vi "gRPC Stream Performance Test.vi"() -> ()   [LabVIEW 2021]
uses:
  streamtest_server/RPC Messages/streamtest_StreamData.ctl
  streamtest_client/RPC Messages/streamtest_StreamData.ctl
  <vilib>/gRPC/LabVIEW gRPC Servicer/Servicer/Servicer.lvclass/Servicer.ctl
  streamtest_server/RPC Service/stream/stream.lvclass
  <vilib>/Platform/TimedLoop/XDataNode/timing_clust.ctl
  <vilib>/Platform/TimedLoop/XDataNode/nitl_modes.ctl
  <vilib>/Platform/TimedLoop/XDataNode/wakeup.ctl
  streamtest_server/RPC Service/stream/stream.lvclass/stream.ctl
  6ba0af29-652a-47d8-b42d-4f43e62654bc.vi
  4033fe76-a443-4ae7-8d99-8cf937cf737c.vi
  <vilib>/gRPC/LabVIEW gRPC Library/Shared/TranslateGrpcError.vi
  grpc perf attempts/_Client obtain occurance.vi
  <vilib>/gRPC/LabVIEW gRPC Library/Server API/Server/Get Server DLL Path.vi
  <vilib>/Utility/error.llb/Error Cluster From Error Code.vi
  <vilib>/Platform/TimedLoop/XDataNode/XDataNode.xnode
  <vilib>/Platform/TimedLoop/XDataNode/XDNodeRunTimeDep.lvlib
  <vilib>/gRPC/LabVIEW gRPC Servicer/Servicer/Servicer.lvclass
  streamtest_server/streamtest_server.lvlib
  streamtest_client/streamtest_client.lvlib
  <vilib>/gRPC/LabVIEW gRPC Library/grpc-lvsupport-release.lvlib
panel:
  out "error out 4":errorcluster
  out "pass 2":bool
  out "avg stream":dbl
  out "Response Data 2":T1
  out "error out 3":errorcluster
  out "Response Data":T1
  out "error out 2":errorcluster
  out "output cluster":T2
  in  "stop":bool
  out "Listening Port":i32
  in  "Server Address":string="localhost:50051"
  in  "Server Certificate File (.crt)":path
  in  "Server Key File (.key)":path
  out "max stream":dbl
  out "pass":bool
  out "error out":errorcluster
  # "This test should be run on RT.  It stresses the communications by constantly creating resource contraints with the low priority sender and the high priority loop. On Windows the priority of the loops cannot be set."
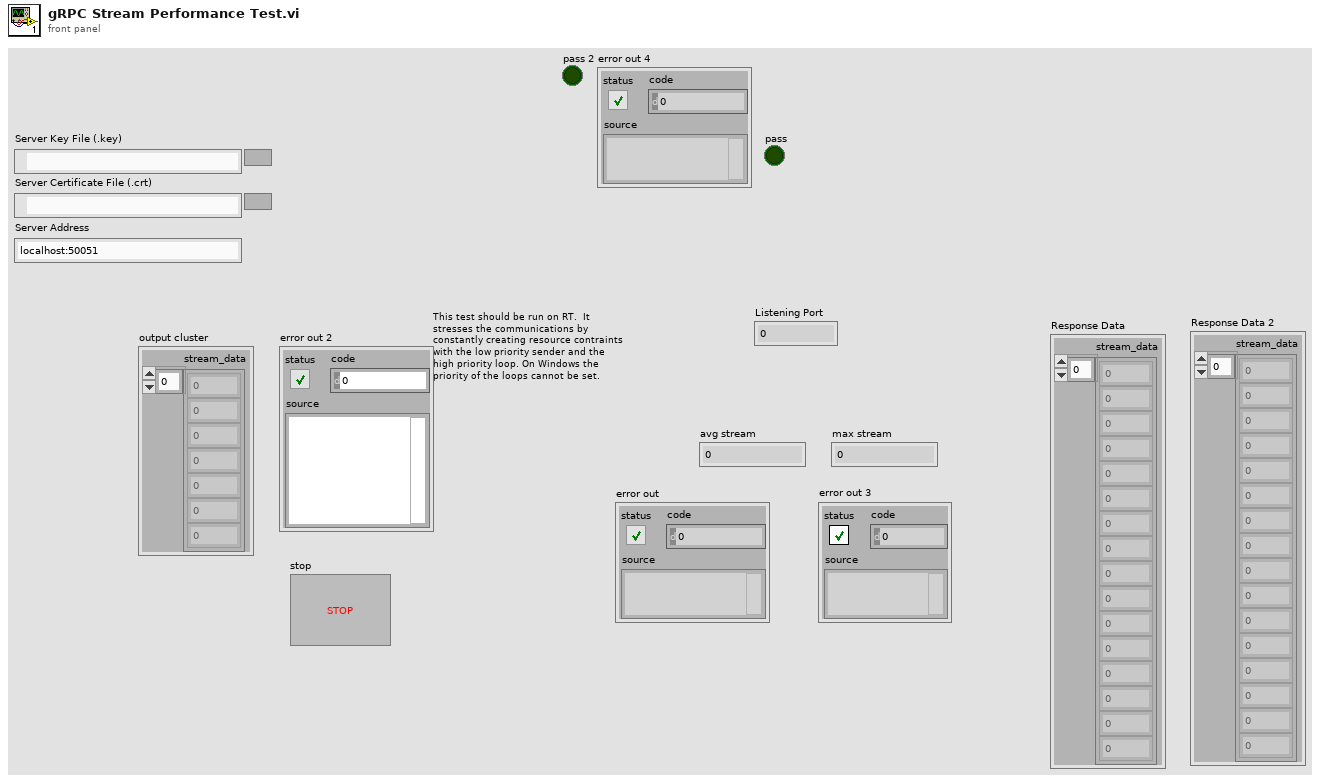
[diagram p1: front panel]
types:
  T1 = typedef "streamtest_client.lvlib/streamtest_StreamData.ctl" = cluster{"stream_data":u8[]}
  T2 = typedef "streamtest_server.lvlib/streamtest_StreamData.ctl" = cluster{"stream_data":u8[]}
  T3 = typedef "grpc-lvsupport-release.lvlib/grpcId.ctl" = u64
  T4 = typedef "Call ID.ctl" = cluster{"Call Id":T3, "occurrence":refnum<k4>}
  T5 = typedef "XDNodeRunTimeDep.lvlib/timing_clust.ctl" = cluster{"Expected End [f-1]":u64, "Actual End [f-1]":u64, "Finished Late? [f-1]":bool, "Expected End [i-1]":u64, "Actual End [i-1]":u64, "Finished Late? [i-1]":bool, "Expected Start [i]":u64, "Actual Start [i]":u64, "Expected Start [f]":u64, "Actual Start [f]":u64, "Source Name":string, "Structure Name":string, "Period":i64, "Deadline":i64, "Offset":i64, "Start":i64, "Priority":i32, "Timeout":i32, "Mode":T6, "Wakeup Reason":T7, "Error":errorcluster, "Source Type":string, "Secondary Source Type":string, "Global End Time":u64, "Global Start Time":u64, "Frame Duration":u64, "Iteration Duration":u64, "Assigned CPU":i32, "I/O Scan Engine Mode":u32}
  T6 = typedef "XDNodeRunTimeDep.lvlib/nitl_modes.ctl" = enum32{"No Change", "Process missed periods, maintain original phase", "Discard missed periods, maintain original phase", "Process missed periods, ignore original phase", "Discard missed periods, ignore original phase"}
  T7 = typedef "XDNodeRunTimeDep.lvlib/wakeup.ctl" = enum32{"Normal", "Aborted", "Asynchronous wakeup", "Timing source error", "Timed loop error", "Timeout"}
  T8 = typedef "streamtest_server.lvlib/stream.lvclass/Server Internal UEs.ctl" = cluster{"stream Send Internal UE":refnum<user-event>}
  T9 = typedef "streamtest_server.lvlib/stream.lvclass/Server gRPC UEs.ctl" = cluster{"stream Send gRPC UE":refnum<user-event>}
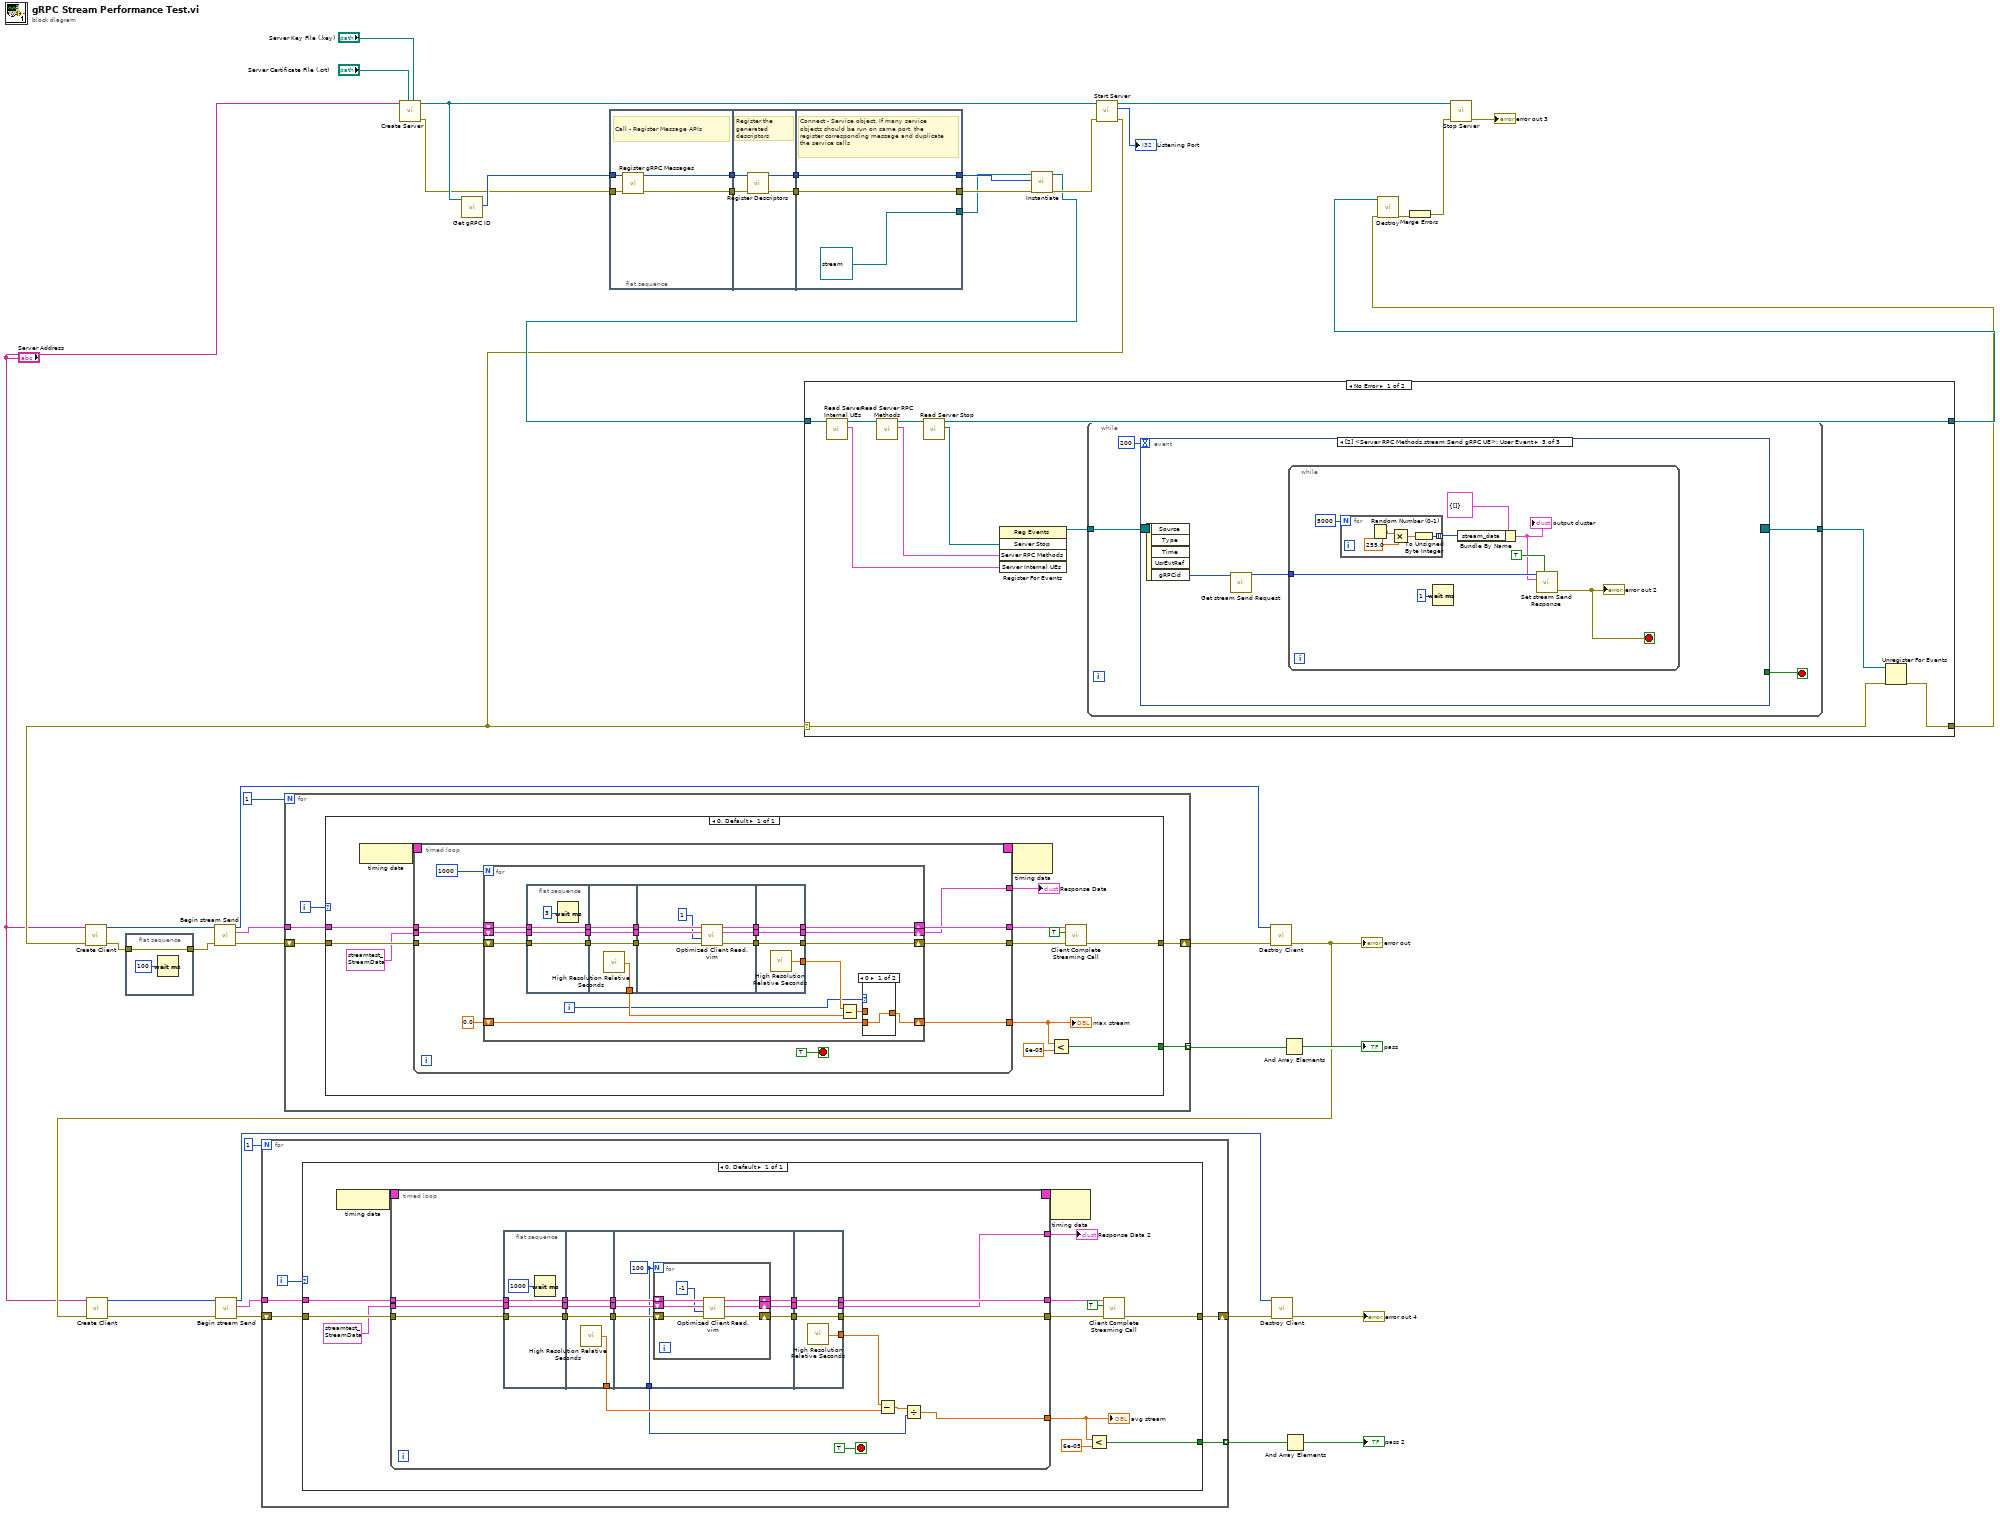
[diagram p0: block diagram]
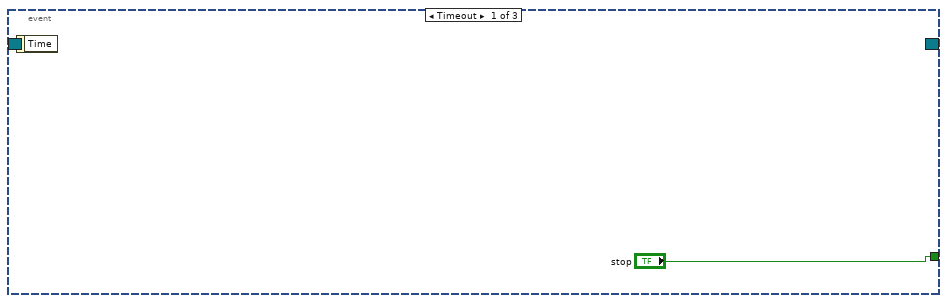
[diagram p2: hidden frame]
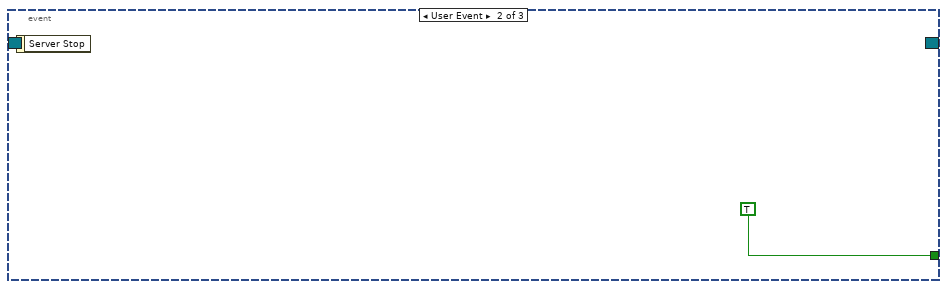
[diagram p3: hidden frame]
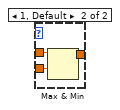
[diagram p5: hidden frame]
diagram:
  n1 = flat-sequence {
    tunnel: w16 -> [w44]
    tunnel: [w44] -> w12
    frame #0 {
      n2 = Wait (ms)(milliseconds to wait=u32 100) -> ()  [unwired: 1 out]
    }
  }
  n3 = call <vilib>:"Create Server.vi"("Server Key File (.key)"="Server Key File (.key)", "Server Certificate File (.crt)"="Server Certificate File (.crt)", "Server Address"="Server Address") -> ("error out"=w26:errorcluster, "gRPC Server out"=w31:refnum<class "Servicer.lvclass">)  [unwired: 7 in]
  n4 = call <vilib>:"Get gRPC ID.vi"("OOP Server in"=w31) -> ("gRPC ID"=w27:T3)  [unwired: 9 in, 1 out]
  n5 = flat-sequence {
    tunnel: w27 -> [w46]
    tunnel: w26 -> [w48]
    tunnel: [w47] -> w39
    tunnel: [w45] -> w38
    tunnel: w39 -> [w51]
    tunnel: w38 -> [w52]
    tunnel: [w49] -> w37
    tunnel: [w50] -> w36
    tunnel: [w54] -> w24
    tunnel: [w55] -> w25
    tunnel: w37 -> [w55]
    tunnel: w36 -> [w54]
    tunnel: [refnum<class "stream.lvclass"> refnum ("streamtest_server.lvlib:stream.lvclass")] -> w23
    frame #0 {
      # "Call - Register Message APIs"
      n6 = call "Register gRPC Messages.vi"("error in (no error)"=w48, "gRPC ID"=w46) -> ("error out"=w47:errorcluster, "gRPC ID Out"=w45:T3)  [unwired: 8 in]
    }
    frame #1 {
      # "Register the generated descriptors"
      n7 = call "Register Descriptors.vi"("error in (no error)"=w51, "gRPC ID"=w52) -> ("error out"=w49:errorcluster, "gRPC ID Out"=w50:T3)  [unwired: 8 in]
    }
    frame #2 {
      # "Connect - Service object. If many service objects should be run on same port, the register corresponding message and duplicate the service calls"
    }
  }
  n8 = call-dynamic "Instantiate.vi"("error in"=w25, "gRPCid"=w24, "iService"=w23) -> ("error out"=w30:errorcluster, "iService"=w22:refnum<class "stream.lvclass">)  [unwired: 7 in]
  n9 = call <vilib>:"Start Server.vi"("error in"=w30, "gRPC Server in"=w31) -> ("error out"=w17:errorcluster, "Listening Port"=→"Listening Port":i32, "gRPC Server out"=w35:refnum<class "Servicer.lvclass">)  [unwired: 7 in]
  n10 = call "Create Client.vi"("error in"=w17, "address"="Server Address") -> ("error out"=w16:errorcluster, "gRPC ID Out"=w19:T3)  [unwired: 8 in]
  n11 = call "Begin stream Send.vi"("error in"=w12, "gRPC ID"=w19) -> ("error out"=w13:errorcluster, "Optimized Streaming"=w18:T4, "gRPC ID out"=w15:T3)  [unwired: 7 in]
  n12 = for {
    N: 1 -> [_]
    tunnel: [w60] -> w41 mode=indexing
    shift-right: [w56] -> w3
    shift-left: w13 -> [w58]
    tunnel: w18 -> [w57]
    i -> [w59]
    n13 = case shown="0, Default" w59 {
      tunnel: [w69] -> w60
      tunnel: w58 -> [w62]
      tunnel: w57 -> [w68]
      tunnel: [w64] -> w56
      frame 0, Default {
        n14 = node-c288() -> (w73:T5)
        n15 = timed-loop {
          timing: w73 -> [_]
          timing-out: [_] -> w72
          tunnel: [w82] -> w67
          tunnel: w68 -> [w75]
          tunnel: [w79] -> w71
          tunnel: w62 -> [w74]
          tunnel: [w78] -> w65
          tunnel: T1 {"stream_data"=[15, 177, 22, 105, 243, 50, 188, 34, 201, 70, 199, 80, 60, 166, 64, 134, 38, 133, 191, 155, 102, 82, 184, 204, 96, 57, 22, 239, 11, 34, 9, 199, 59, 124, 146, 252, 83, 47, 53, 8, 172, 34, 179, 226, 220, 102, 247, 239, 92, 187, 120, 214, 121, 133, 209, 198, 116, 175, 147, 100, 229, 131, 147, 4, 66, 95, 150, 24, 239, 3, 89, 131, 33, 53, 108, 163, 198, 156, 165, 92, 104, 234, 223, 105, 240, 66, 39, 28, 180, 10, 135, 177, 27, 124, 48, 109, 168, 71, 127, 64]} ("Response Data") -> [w77]
          tunnel: [w76] -> w63
          stop <- TRUE stop-if-true
          n16 = for {
            N: 1000 -> [_]
            shift-right: [w94] -> w82
            shift-left: w74 -> [w102]
            shift-right: [w96] -> w79
            shift-left: 0.0 -> [w97]
            shift-right: [w92] -> w78
            shift-left: w75 -> [w101]
            shift-right: [w88] -> w76
            shift-left: w77 -> [w84]
            i -> [w95]
            n17 = flat-sequence {
              tunnel: w101 -> [w111]
              tunnel: w102 -> [w112]
              tunnel: [w112] -> w90
              tunnel: [w111] -> w89
              tunnel: [w109] -> w85
              tunnel: w84 -> [w109]
              tunnel: [w116] -> w104
              tunnel: [w115] -> w99
              tunnel: [w114] -> w103
              tunnel: w90 -> [w116]
              tunnel: w89 -> [w114]
              tunnel: [w113] -> w86
              tunnel: w85 -> [w113]
              tunnel: w104 -> [w123]
              tunnel: w103 -> [w121]
              tunnel: [w122] -> w93
              tunnel: [w119] -> w91
              tunnel: [w118] -> w87
              tunnel: w86 -> [w120]
              tunnel: [w127] -> w100
              tunnel: [w126] -> w94
              tunnel: w93 -> [w126]
              tunnel: [w125] -> w92
              tunnel: w91 -> [w125]
              tunnel: [w124] -> w88
              tunnel: w87 -> [w124]
              frame #0 {
                n18 = Wait (ms)(milliseconds to wait=u32 3) -> ()  [unwired: 1 out]
              }
              frame #1 {
                n19 = call <vilib>:"High Resolution Relative Seconds.vi"() -> ("relative seconds"=w115:dbl)
              }
              frame #2 {
                n20 = call "Optimized Client Read.vim"("error in"=w123, "timeout ms (-1)"=1 ("ms timeout (-1)"), "Response Type"=w120, "Optimized Streaming in"=w121) -> ("error out"=w122:errorcluster, "Response Data"=w118:T1, "Optimized Streaming out"=w119:T4)  [unwired: 3 in, 2 out]
              }
              frame #3 {
                n21 = call <vilib>:"High Resolution Relative Seconds.vi"() -> ("relative seconds"=w127:dbl)
              }
            }
            n22 = Subtract(x=w100, y=w99) -> (x-y=w98:dbl)
            n23 = case shown="0" w95 {
              tunnel: w98 -> [_ w108]
              tunnel: w97 -> [w105 w107]
              tunnel: [w105 w106] -> w96
              frame 0 {
              }
              frame 1, Default {
                n24 = Max & Min(x=w108, y=w107) -> (max(x,y)=w106:dbl)  [unwired: 1 out]
              }
            }
          }
        }
        "max stream" <- w71
        "Response Data" <- w63
        n25 = node-c288(w72) -> ()  [unwired: 1 out]
        n26 = Less?(x=w71, y=6e-05) -> (x < y?=w69:bool)
        n27 = call <vilib>:"Client Complete Streaming Call.vi"("error in"=w67, "Cancel All Reads (T)"=TRUE ("Cancel All Reads (F)"), "Optimized Streaming in"=w65) -> ("error out"=w64:errorcluster)  [unwired: 7 in, 1 out]
      }
    }
  }
  "error out" <- w3
  n28 = call "Create Client.vi"("error in"=w3, "address"="Server Address") -> ("error out"=w1:errorcluster, "gRPC ID Out"=w7:T3)  [unwired: 8 in]
  n29 = call "Begin stream Send.vi"("error in"=w1, "gRPC ID"=w7) -> ("error out"=w11:errorcluster, "Optimized Streaming"=w8:T4, "gRPC ID out"=w10:T3)  [unwired: 7 in]
  n30 = for {
    N: 1 -> [_]
    tunnel: [w136] -> w5 mode=indexing
    shift-right: [w132] -> w9
    shift-left: w11 -> [w134]
    tunnel: w8 -> [w133]
    i -> [w135]
    n31 = case shown="0, Default" w135 {
      tunnel: [w145] -> w136
      tunnel: w134 -> [w138]
      tunnel: w133 -> [w144]
      tunnel: [w140] -> w132
      frame 0, Default {
        n32 = node-c288() -> (w149:T5)
        n33 = timed-loop {
          timing: w149 -> [_]
          timing-out: [_] -> w148
          tunnel: [w169] -> w143
          tunnel: w144 -> [w165]
          tunnel: [w150] -> w147
          tunnel: w138 -> [w164]
          tunnel: [w168] -> w141
          tunnel: T1 {"stream_data"=[15, 177, 22, 105, 243, 50, 188, 34, 201, 70, 199, 80, 60, 166, 64, 134, 38, 133, 191, 155, 102, 82, 184, 204, 96, 57, 22, 239, 11, 34, 9, 199, 59, 124, 146, 252, 83, 47, 53, 8, 172, 34, 179, 226, 220, 102, 247, 239, 92, 187, 120, 214, 121, 133, 209, 198, 116, 175, 147, 100, 229, 131, 147, 4, 66, 95, 150, 24, 239, 3, 89, 131, 33, 53, 108, 163, 198, 156, 165, 92, 104, 234, 223, 105, 240, 66, 39, 28, 180, 10, 135, 177, 27, 124, 48, 109, 168, 71, 127, 64]} ("Response Data") -> [w167]
          tunnel: [w166] -> w139
          stop <- TRUE stop-if-true
          n34 = flat-sequence {
            tunnel: w165 -> [w173]
            tunnel: w164 -> [w174]
            tunnel: [w174] -> w163
            tunnel: [w173] -> w162
            tunnel: [w171] -> w161
            tunnel: w167 -> [w171]
            tunnel: [w178] -> w160
            tunnel: [w177] -> w153
            tunnel: [w176] -> w159
            tunnel: w163 -> [w178]
            tunnel: w162 -> [w176]
            tunnel: [w175] -> w158
            tunnel: w161 -> [w175]
            tunnel: w160 -> [w185]
            tunnel: w159 -> [w183]
            tunnel: [w184] -> w157
            tunnel: [w181] -> w156
            tunnel: [w180] -> w155
            tunnel: w158 -> [w182]
            tunnel: [w179] -> w151
            tunnel: [w196] -> w154
            tunnel: [w195] -> w169
            tunnel: w157 -> [w195]
            tunnel: [w194] -> w168
            tunnel: w156 -> [w194]
            tunnel: [w193] -> w166
            tunnel: w155 -> [w193]
            frame #0 {
              n35 = Wait (ms)(milliseconds to wait=u32 1000) -> ()  [unwired: 1 out]
            }
            frame #1 {
              n36 = call <vilib>:"High Resolution Relative Seconds.vi"() -> ("relative seconds"=w177:dbl)
            }
            frame #2 {
              w179 = 100
              n37 = for {
                N: w179 -> [_]
                shift-right: [w191] -> w184
                shift-left: w185 -> [w192]
                shift-right: [w188] -> w181
                shift-left: w183 -> [w190]
                shift-right: [w187] -> w180
                shift-left: w182 -> [w189]
                n38 = call "Optimized Client Read.vim"("error in"=w192, "timeout ms (-1)"=-1 ("ms timeout (-1)"), "Response Type"=w189, "Optimized Streaming in"=w190) -> ("error out"=w191:errorcluster, "Response Data"=w187:T1, "Optimized Streaming out"=w188:T4)  [unwired: 3 in, 2 out]
              }
            }
            frame #3 {
              n39 = call <vilib>:"High Resolution Relative Seconds.vi"() -> ("relative seconds"=w196:dbl)
            }
          }
          n40 = Subtract(x=w154, y=w153) -> (x-y=w152:dbl)
          n41 = Divide(x=w152, y=w151) -> (x/y=w150:dbl)
        }
        "avg stream" <- w147
        "Response Data 2" <- w139
        n42 = node-c288(w148) -> ()  [unwired: 1 out]
        n43 = Less?(x=w147, y=6e-05) -> (x < y?=w145:bool)
        n44 = call <vilib>:"Client Complete Streaming Call.vi"("error in"=w143, "Cancel All Reads (T)"=TRUE ("Cancel All Reads (F)"), "Optimized Streaming in"=w141) -> ("error out"=w140:errorcluster)  [unwired: 7 in, 1 out]
      }
    }
  }
  "error out 4" <- w9
  n45 = case shown="No Error" w17 {
    selector: w17 -> [w205 w233]
    tunnel: [w204 w233] -> w20
    tunnel: [w202 w232] -> w21
    tunnel: w22 -> [w211 w232]
    frame No Error {
      n46 = call "Read Server Internal UEs.vi"("SignalGeneratorService in"=w211) -> ("Server Internal UEs"=w209:T8, "SignalGeneratorService out"=w210:refnum<class "stream.lvclass">)  [unwired: 8 in, 1 out]
      n47 = call "Read Server RPC Methods.vi"("SignalGeneratorService in"=w210) -> ("Server RPC Methods"=w203:T9, "SignalGeneratorService out"=w208:refnum<class "stream.lvclass">)  [unwired: 8 in, 1 out]
      n48 = call-dynamic "Read Server Stop.vi"("iService in"=w208) -> ("Server Stop"=w201:refnum<user-event>, "iService out"=w202:refnum<class "stream.lvclass">)  [unwired: 8 in, 1 out]
      n49 = register-events(w201, w203, w209) -> (reference out=w207:refnum<event-registration>)  [unwired: 2 in, 1 out]
      n50 = while {
        tunnel: w207 -> [w215]
        tunnel: [w213] -> w206
        stop <- w214 stop-if-true
        n51 = event "RPC Methods Event Structure" shown="[2] <Server RPC Methods.stream Send gRPC UE>: User Event" {
          selector: w215 -> [_ _ _]
          dyn-events: [_ _ _] -> w213
          timeout: 200 -> [_ _ _]
          tunnel: ["stop" TRUE _] -> w214
          event Timeout {
            n52 = event-data() -> ()  [unwired: 1 in, 1 out]
          }
          event User Event {
            n53 = event-data() -> ()  [unwired: 1 in, 1 out]
          }
          event User Event {
            n54 = event-data() -> ("gRPCid"=w219:T3)  [unwired: 1 in, 4 out]
            n55 = call "Get stream Send Request.vi"("gRPCid"=w219) -> ("gRPCid out"=w218:T3)  [unwired: 8 in, 2 out]
            n56 = while {
              tunnel: w218 -> [w227]
              stop <- w220 stop-if-true
              n57 = for {
                N: 5000 -> [_]
                tunnel: [w228] -> w223 mode=indexing
                n58 = Random Number (0-1)() -> (number: 0 to 1=w231:dbl)
                n59 = Multiply(x=w231, y=255.0) -> (x*y=w229:dbl)
                n60 = To Unsigned Byte Integer(number=w229) -> (unsigned 8bit integer=w228:u8)
              }
              n61 = Wait (ms)(milliseconds to wait=u32 1) -> ()  [unwired: 1 out]
              n62 = Bundle By Name(cluster=T2 {"stream_data"=[]} ("Message Data"), "stream_data"=w223) -> (w222:T2)
              "output cluster" <- w222
              n63 = call "Set stream Send Response.vi"("Streaming? (F)"=TRUE, "Message Data"=w222, "gRPCid in"=w227) -> ("error out"=w220:errorcluster)  [unwired: 8 in]
              "error out 2" <- w220
            }
          }
        }
      }
      n64 = Unregister For Events(event registration refnum=w206, error in=w205) -> (error out=w204:errorcluster)
    }
    frame Error {
    }
  }
  n65 = call "Destroy Client.vi"("error in"=w3, "gRPC ID"=w15) -> ()  [unwired: 9 in, 1 out]
  n66 = call "Destroy Client.vi"("error in"=w9, "gRPC ID"=w10) -> ()  [unwired: 9 in, 1 out]
  n67 = And Array Elements(Boolean array=w41) -> (logical AND=→"pass":bool)
  n68 = And Array Elements(Boolean array=w5) -> (logical AND=→"pass 2":bool)
  n69 = call-dynamic "Destroy.vi"("error in (no error)"=w20, "SignalGeneratorService in"=w21) -> ("error out"=w29:errorcluster)  [unwired: 8 in, 1 out]
  n70 = Merge Errors(w29) -> (w28:errorcluster)
  n71 = call <vilib>:"Stop Server.vi"("error in"=w28, "gRPC Server in"=w35) -> ("error out"=→"error out 3":errorcluster)  [unwired: 9 in]
